vi "AppendErrors.vi"   [LabVIEW 2017, in "GPError.lvlib"]
doc: "Appends <B>Error to append</B> to <B>Error in</B>.\n\nAppending errors preserves the contents of the two error clusters opposed to merging errors (with the built-in 'Merge Errors' function) which only keeps the highest priority error and scraps the rest. Appending errors maintains all error information inside the Source string of a single error cluster. Built-in, overridden and custom errors are supported.\n\nUse the SplitAppended function to split an appended error cluster into an array of individual error clusters.\n\nOnly errors and warnings are appended, any 'No error' is skipped.\n\nThe optional <B>Only append if new?</B> will, if set to True (which is the default setting), make this VI test if <B>Error to append</B> is already present in <B>Error in</B>. If that is the case (possibly as an earlier appended error) then no new append will occur. This feature is valuable if you append errors in a loop and risk encountering the same error over and over again, but you don't want to keep piling up all new copies of the same error. Set <B>Only append if new?</B> to False to append unconditionally.\n\nThis function considers two errors equal only if their code, status, source and description fields are all identical. Two errors that differ only in timestamp are considered equal as well however, the one already present in <B>Error in</B> staying put.\n\nThis VI might change the order of the appended errors, as it will always seek to move at least one error in front of any warnings in the appended error collection. This is to avoid any of the built-in LabVIEW functions wrongfully overwriting an appended error with its own error, which it will if a warning is the top-most value in the appended error collection.\n\nThis VI is polymorphic, accepting either a single error or an array of errors to append.\n\nSteen Schmidt\nGPower"
uses:
  GPError.lvlib
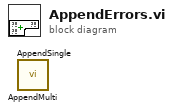
[diagram p0: block diagram]
diagram:
  n1 = call "AppendMulti.vi"() -> ()  [unwired: 11 in, 1 out]
  n2 = call "AppendSingle.vi"() -> ()  [unwired: 11 in, 1 out]
